vi "MeanderCtrl_3d_StageRefs.vi"(0 "QueuesRef":T1, 1 "MotionStageRefs":refnum<queue>, 2 "AppsRef":refnum<queue>, 3 "SecondaryVI_Ref":refnum<vi>, 4 "SecondaryParams":variant[](array[variant]), 5 "start/end points":cluster{dbl, dbl, dbl}[][](array[cluster]), 9 "Laser_Ctrl":bool, 11 "error in":errorcluster, 12 "HighSpeed":dbl=5.0, 13 "ScanSpeed":dbl=0.1, 14 "KeepStill":u32) -> (6 "Interupted":bool, 8 "Actual_Line#":i32, 15 "error out":errorcluster)   [LabVIEW 2013]
uses:
  ControlDef/QueueRefs.ctl
  ControlDef/LaserCtrl_Method.ctl
  ControlDef/States-AToF.ctl
  <instrlib>/AnalogDiscSDKLv/VIs/DWF_CtrlQueue.ctl
  <instrlib>/AnalogDiscSDKLv/VIs/DWF_State.ctl
  <instrlib>/ESP300/Public/Data/ESP300_State.ctl
  <instrlib>/DG535/Command/DG535_States.ctl
  Hardware/BNC(QuantumComposers)/BNC_States.ctl
  Hardware/FemtoLaser(Legacy)/Laser_Status.ctl
  Hardware/DAQmx(Legacy)/DAQmx_Status.ctl
  ControlDef/Signal.ctl
  ProcessMethods/SignalAverager/ProcessStates.ctl
  Files/WriterState.ctl
  Files/Signal_Segment.ctl
  ControlDef/ProcessingMode.ctl
  Hardware/EPM2000(Legacy)/EPM2K_Status.ctl
  <instrlib>/AnalogDiscSDKLv/VIs/DWF_Signal.ctl
  MeanderLoopState.ctl
  <instrlib>/ESP300/Public/Data/ESP30x_Data.ctl
  <instrlib>/Micos_uic/Public/Data/Micos_Data.ctl
  ControlDef/PauseMeander.vi
  <instrlib>/ESP300/ESP300.lvlib
  <instrlib>/Micos_uic/Micos_uic.lvlib
  <instrlib>/DG535/SRS_DG535_Lib.lvlib
  <userlib>/Utility/ErrorLog_lib.lvlib
  <instrlib>/AnalogDiscSDKLv/AnalogDiscSDKLv.lvlib
panel:
  out "InnerIter.":i32
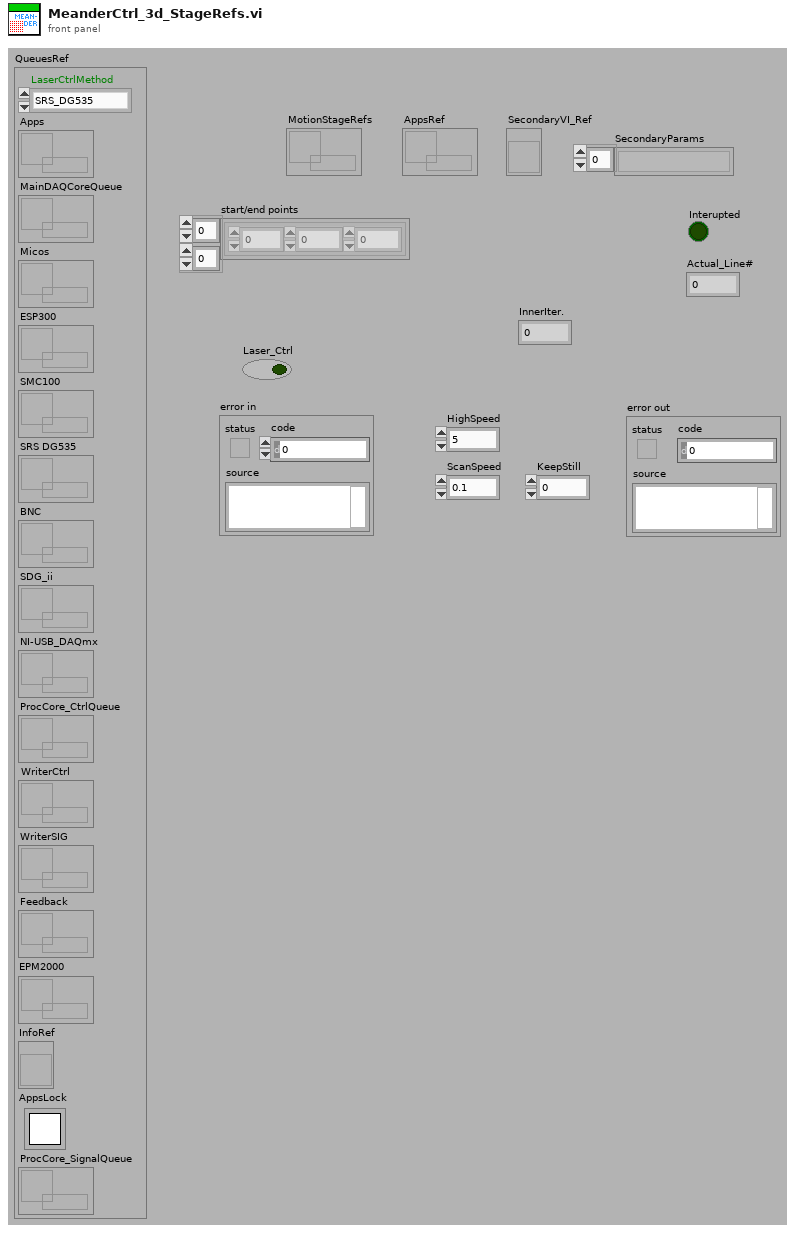
[diagram p1: front panel]
types:
  T1 = typedef "QueueRefs.ctl" = cluster{"LaserCtrlMethod":T2, "Apps":refnum<queue>, "MainDAQCoreQueue":refnum<queue>, "Micos":refnum<queue>, "ESP300":refnum<queue>, "SMC100":refnum<queue>, "SRS DG535":refnum<queue>, "BNC":refnum<queue>, "SDG_ii":refnum<queue>, "NI-USB_DAQmx":refnum<queue>, "ProcCore_CtrlQueue":refnum<queue>, "WriterCtrl":refnum<queue>, "WriterSIG":refnum<queue>, "Feedback":refnum<queue>, "EPM2000":refnum<queue>, "InfoRef":refnum<vi>, "AppsLock":T3, "ProcCore_SignalQueue":refnum<queue>}
  T2 = typedef "LaserCtrl_Method.ctl" = enum16{"SRS_DG535", "BNC", "SDG_II"}
  T3 = typedef "Semaphore RefNum" = refnum<k1>
  T4 = typedef "States-AToF.ctl" = enum16{"Initialize", "Idle", "CalcMzArray", "Meander_SGL_MCS", "Meander_MCS", "CleanSurface", "Meander_Npt", "Meander_SGL_Npt", "KnifeEdgeExpt", "KnifeEdgeExpt_Npt", "Imaging_Micos", "Imaging_ESP", "DepthProfiling", "Set_2PulseDelay", "DelayScan", "PeakSearch", "ExportOrigin", "Save Settings", "Load Settings", "Save as Default", "Load Default", "EnergyCalibration", "Quit", "Interrupted_Stop", "Quit_SubProgram", "StepMove_Joystick", "ContMove_Joystick", "Stop_Joystick", "Check_AppsLock", "Return_Status", "DepthProfile_RT", "UpdateInstruStates", "InstruOptimizer_static", "instruOptimizer_dynamic"}
  T5 = typedef "MeanderLoopState.ctl" = enum16{"Pre-Start", "Send-loginfo", "SetHighVelocity", "MoveToLineStart", "SetSecondaryParams", "WaitStartReady", "UpdateStartPosition", "StartOfLine", "SetLowVelocity", "MoveToLineEnd", "StartLaser_move", "WaitScanFinish", "StartLaser_still", "KeepStill", "StopLaser", "EndOfLine", "CheckPause", "Exit", "RestoreVelocity", "Pause", "Quit"}
  T6 = typedef "ESP300.lvlib/ESP300_State.ctl" = cluster{"State":enum16{"Initialize", "SetDefaultConfig", "Close", "Quit", "Identify", "MoveAbs", "MoveAbs_all", "MoveRel", "MoveRel_all", "STOP", "Origin/Home", "WaitStop", "QueryStatus", "UpdateXPos", "UpdateAll", "SetVelocity", "SetAcceleration", "ClearErr", "LogMessage", "MotorEnable(1)", "EnableAxis", "JoyStick", "GetVelocity", "GetAcceleration", "SendCmd", "SetSoftLimits", "Beep", "_SettingReturn", "SoftReset"}, "Params.":variant}
  T7 = typedef "ESP300.lvlib/ESP30x_Data.ctl" = cluster{"Position":dbl[], "Velocity":dbl[], "Acceleration":dbl[], "Moving":bool, "Simulation":bool, "tickcount_mov":u32, "tickcount_pos":u32, "NumOfAxis":i32, "Initialized":bool, "CommPort":refnum<visa-resource-name>, "Range":dbl[][], "Serial Configuration":cluster{"Baud Rate":u32, "Parity":u16, "Data Bits":u16, "Stop Bits":u16, "Flow Control":u16}, "MotorDisabled":refnum<vi>}
  T8 = typedef "Signal.ctl" = cluster{"Command":T9, "Params":variant}
  T9 = typedef "ProcessStates.ctl" = enum16{"Initialize", "Normal", "Display", "Write2Buffer", "CalcMzArray", "StartSave", "StopSave", "ConfigChanged", "EndOfLine", "SetFilterParams", "SetGraphsEnable", "SetAcquisitionParams", "ChangeDisplayIncrement", "ChangeRepRate", "SetWriterRef", "Quit", "StartOfLine"}
  T10 = typedef "Laser_Status.ctl" = cluster{"State":enum16{"Initialize", "Idle/Update", "Configure", "Turn On", "Tun OFF", "Continuous", "Single Shot", "ManualTrigger", "Close", "Quit"}, "Parameter":dbl}
  T11 = typedef "BNC_States.ctl" = cluster{"State":enum16{"Initialize", "Set System", "Set C-Input", "Set C-Mode", "Set C-Output", "Set C-Enable", "Manl_Trig", "Run", "Stop", "Query C Number", "Close", "Quit"}, "Para.":variant}
  T12 = typedef "SRS_DG535_Lib.lvlib/DG535_States.ctl" = cluster{"State":enum16{"Initialize", "Set Trigger", "Set Output", "Set Delay", "Manl_Trig", "Run", "Stop", "Close", "Quit"}, "Para.":variant}
  T13 = typedef "Micos_uic.lvlib/Micos_Data.ctl" = cluster{"Position":dbl[], "Velocity":dbl[], "Acceleration":dbl[], "Moving":bool, "Simulation":bool, "tickcount_mov":u32, "tickcount_pos":u32, "NumOfAxis":i32, "Initialized":bool, "CommPort":refnum<visa-resource-name>, "Range":dbl[][], "Serial Configuration":cluster{"Baud Rate":u32, "Parity":u16, "Data Bits":u16, "Stop Bits":u16, "Flow Control":u16}, "MotorDisabled":refnum<vi>}
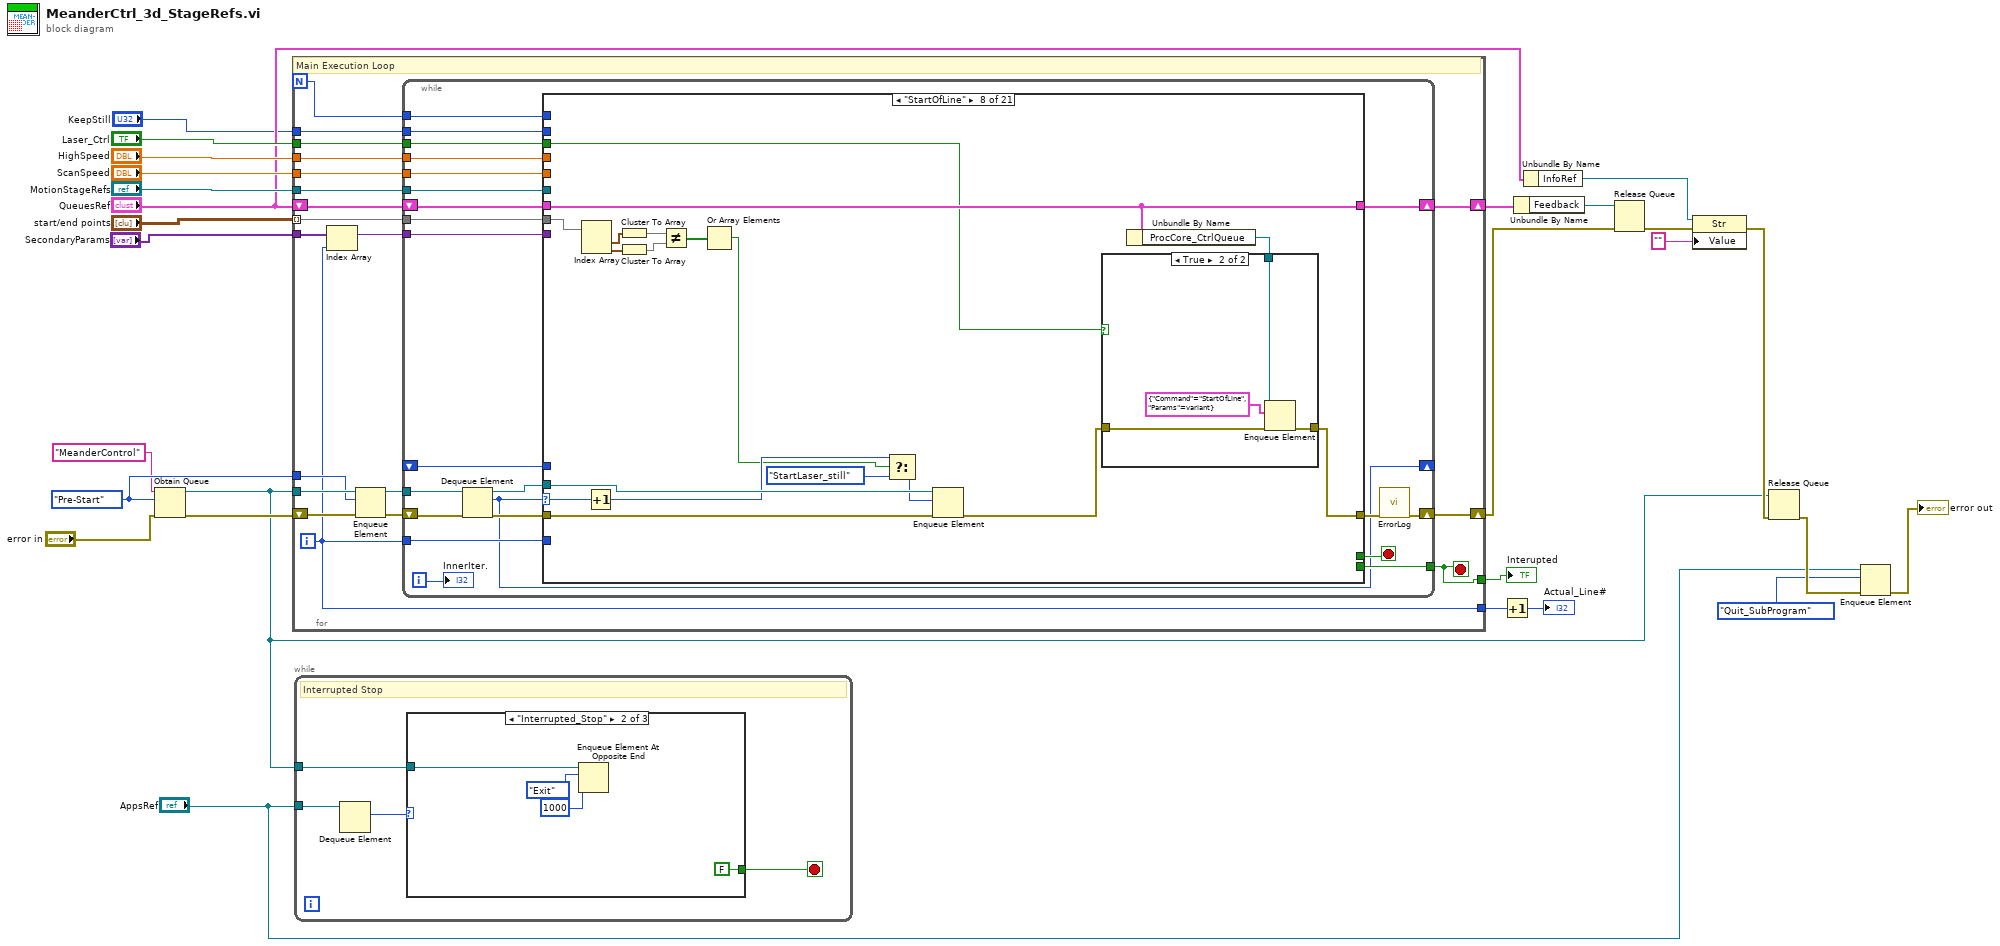
[diagram p0: block diagram]
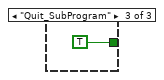
[diagram p3: hidden frame]
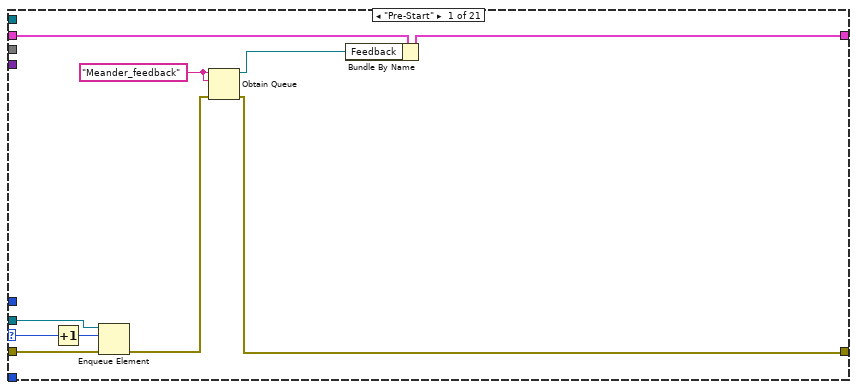
[diagram p4: hidden frame]
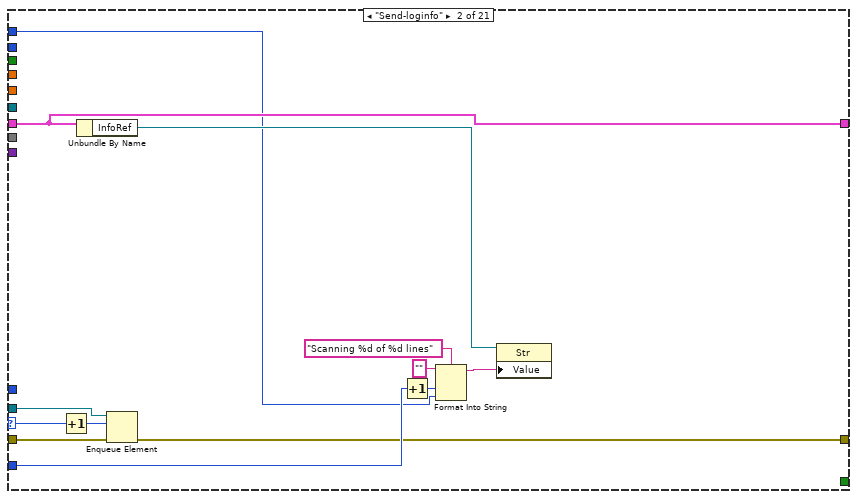
[diagram p5: hidden frame]
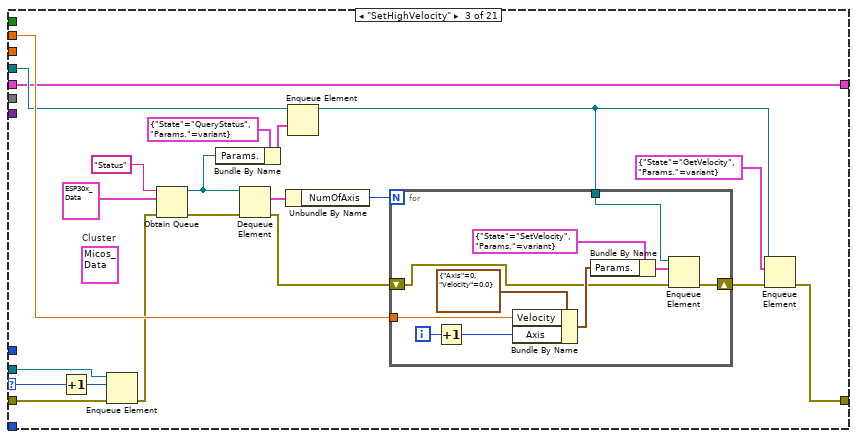
[diagram p6: hidden frame]
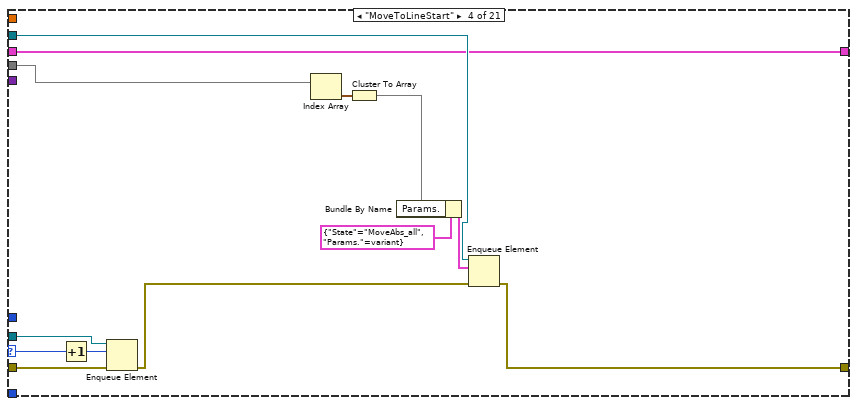
[diagram p7: hidden frame]
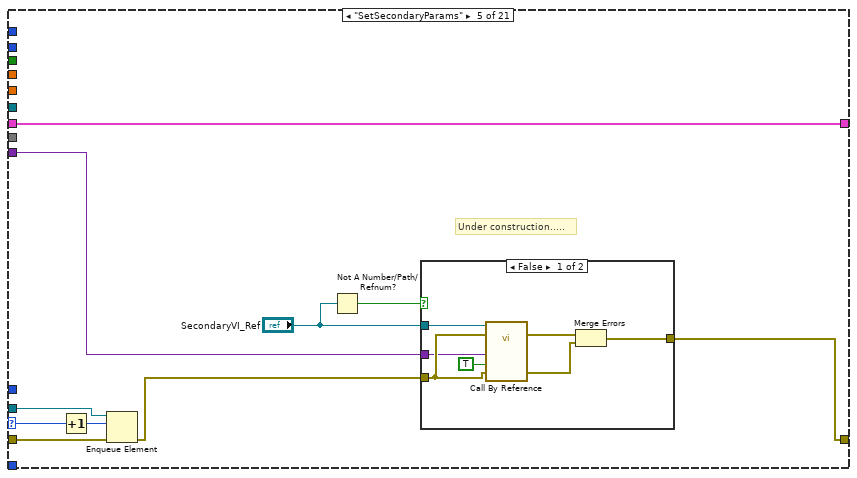
[diagram p8: hidden frame]
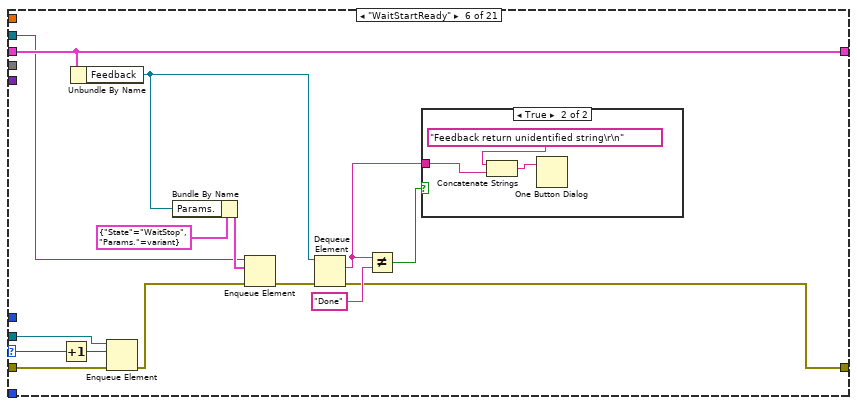
[diagram p10: hidden frame]
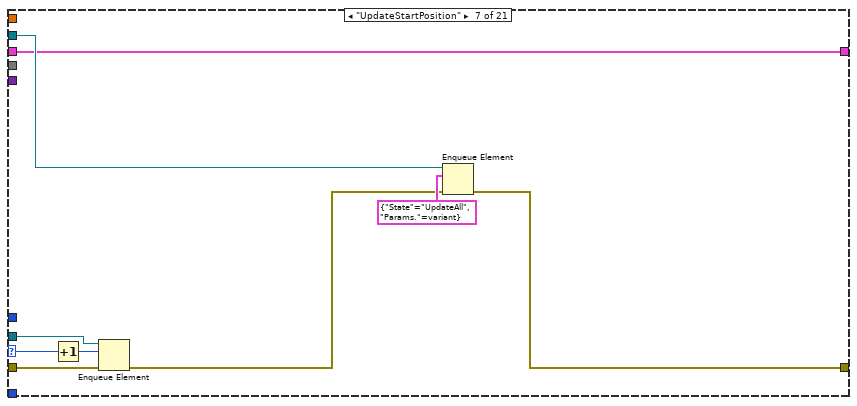
[diagram p12: hidden frame]
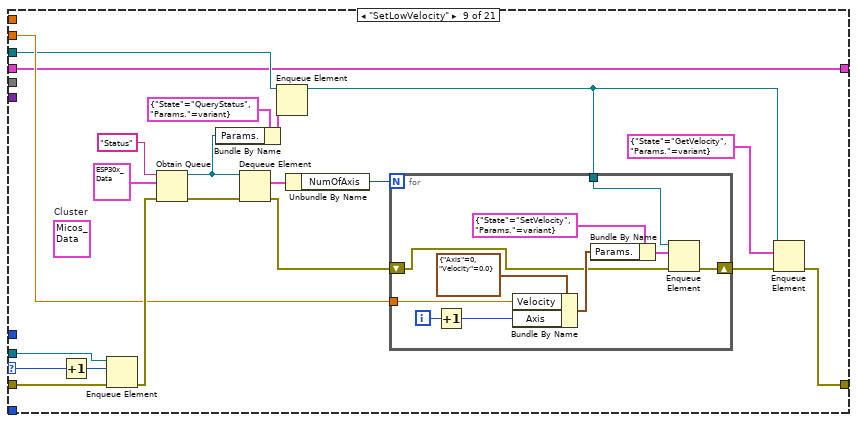
[diagram p14: hidden frame]
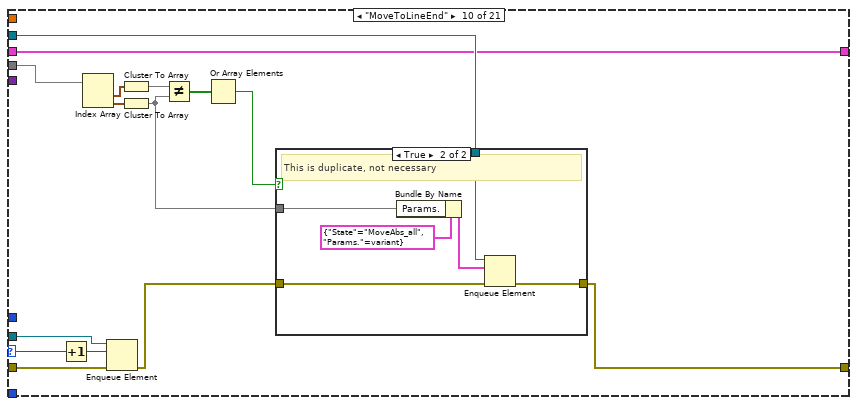
[diagram p15: hidden frame]
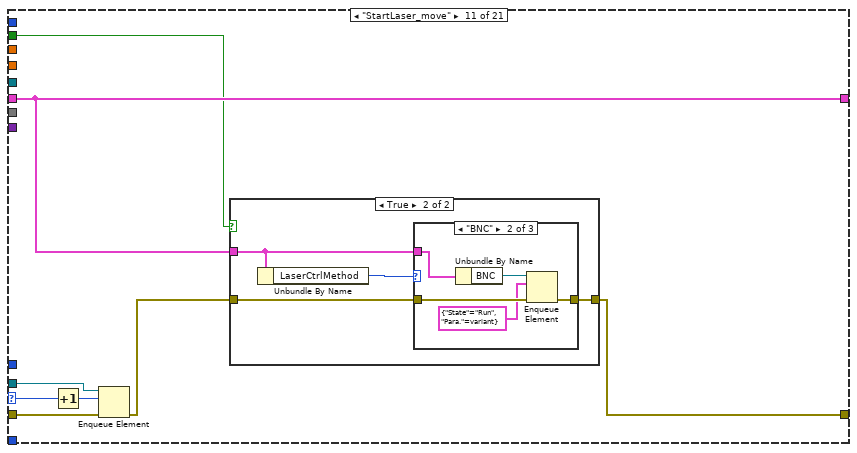
[diagram p17: hidden frame]
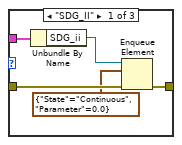
[diagram p19: hidden frame]
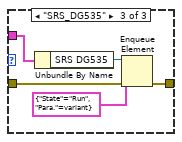
[diagram p20: hidden frame]
diagram:
  w15 = MeanderLoopState."Pre-Start"
  n1 = Obtain Queue(name (unnamed)="MeanderControl", element data type=w15, error in (no error)="error in") -> (queue out=w12:refnum<queue>, error out=w18:errorcluster)  [unwired: 2 in, 1 out]
  n2 = for {
    N -> [w35]
    tunnel: "MotionStageRefs" -> [w45]
    tunnel: "ScanSpeed" -> [w43]
    tunnel: "HighSpeed" -> [w42]
    tunnel: w12 -> [w41]
    tunnel: "start/end points" -> [w40] mode=indexing
    tunnel: "Laser_Ctrl" -> [w39]
    tunnel: [w28] -> w22
    shift-right: [w38] -> w1
    shift-left: w18 -> [w37]
    tunnel: [w36] -> w16
    tunnel: w15 -> [w33]
    shift-right: [w32] -> w3
    shift-left: "QueuesRef" -> [w44]
    tunnel: "KeepStill" -> [w31]
    tunnel: "SecondaryParams" -> [w30]
    i -> [w28]
    stop <- w36 stop-if-true
    # "Main Execution Loop"
    n3 = Index Array(array=w30, index=w28) -> (element=w29:variant)
    n4 = Enqueue Element(queue=w41, element=w33) -> (queue out=w34:refnum<queue>)  [unwired: 2 in, 2 out]
    n5 = while {
      tunnel: w45 -> [w67]
      tunnel: w43 -> [w65]
      tunnel: w42 -> [w64]
      tunnel: w34 -> [w63]
      tunnel: w28 -> [w61]
      shift-right: [w47] -> w38
      shift-left: w37 -> [w58]
      tunnel: w40 -> [w56]
      tunnel: w39 -> [w55]
      shift-right: [w46] -> _
      shift-left: _ -> [w54]
      tunnel: [w53] -> w36
      tunnel: w35 -> [w52]
      shift-right: [w51] -> w32
      shift-left: w44 -> [w66]
      tunnel: w31 -> [w50]
      tunnel: w29 -> [w48]
      i -> [w49]
      stop <- w62 stop-if-true
      n6 = Dequeue Element(queue=w63, error in (no error)=w58) -> (queue out=w60:refnum<queue>, element=w46:T5, error out=w59:errorcluster)  [unwired: 1 in, 1 out]
      n7 = case shown="\"StartOfLine\"" w46 {
        selector: w46 -> [w77 w90 w111 w134 w144 w167 w179 w197 w223 w248 w263 w298 w312 w340 w365 _ _ _ _ _ _]
        tunnel: w67 -> [_ _ w97 w123 _ w153 w174 _ w210 w240 _ w284 _ _ _ _ w410 _ w468 _ _]
        tunnel: w66 -> [w71 w85 w96 w122 w140 w165 w171 w194 w209 w239 w259 w296 w304 w336 w360 w392 w409 w440 w461 w470 w500]
        tunnel: w65 -> [_ _ _ _ _ _ _ _ w211 _ _ _ _ _ _ _ _ _ _ _ _]
        tunnel: w64 -> [_ _ w107 _ _ _ _ _ _ _ _ _ _ _ _ _ w421 _ _ _ _]
        tunnel: [_ _ _ _ _ _ _ _ _ _ _ _ _ _ _ _ w400 TRUE _ _ w499] -> w62
        tunnel: w61 -> [_ w83 _ _ _ _ _ _ _ _ _ _ _ _ _ _ _ _ _ _ _]
        tunnel: w60 -> [w72 w82 w109 w132 w142 w164 w177 w196 w221 w246 w261 w295 w310 w333 w363 w394 w407 w439 w458 w474 _]
        tunnel: w59 -> [w75 w81 w108 w131 w141 w163 w176 w195 w220 w245 w260 w294 w309 w338 w362 w393 w406 w442 w469 w477 w498]
        tunnel: [w73 w80 w91 w124 w138 w154 w172 w191 w204 w242 w256 w285 w302 w337 w358 w389 w412 w438 _ w476 w498] -> w57
        tunnel: w56 -> [_ _ _ w128 _ _ _ w183 _ w244 _ _ _ _ _ _ _ _ _ _ _]
        tunnel: w55 -> [_ _ _ _ _ _ _ w190 _ _ w258 _ w308 _ w361 w388 _ _ _ _ _]
        tunnel: w54 -> [_ _ _ _ _ _ _ _ _ _ _ _ _ _ _ _ w404 _ _ _ _]
        tunnel: [_ _ _ _ _ _ _ _ _ _ _ _ _ _ _ _ w401 w441 _ _ w499] -> w53
        tunnel: w52 -> [_ w78 _ _ _ _ _ _ _ _ _ _ _ _ _ _ _ _ _ _ _]
        tunnel: [w70 w85 w96 w122 w140 w165 w171 w194 w209 w239 w259 w296 w304 w336 w360 w392 w409 w440 w461 w470 w500] -> w51
        tunnel: w50 -> [_ _ _ _ _ _ _ _ _ _ _ _ w307 w335 _ _ _ _ _ _ _]
        tunnel: w48 -> [_ _ _ _ w135 _ _ _ _ _ _ _ _ _ _ _ _ _ _ _ _]
        frame "Pre-Start" {
          w68 = "Meander_feedback" ("name (unnamed)")
          n8 = Increment(x=w77) -> (x+1=w76:T5)
          n9 = Enqueue Element(queue=w72, element=w76, error in (no error)=w75) -> (error out=w74:errorcluster)  [unwired: 1 in, 2 out]
          n10 = Obtain Queue(name (unnamed)=w68, element data type=w68, error in (no error)=w74) -> (queue out=w69:refnum<queue>, error out=w73:errorcluster)  [unwired: 2 in, 1 out]
          n11 = Bundle By Name(cluster=w71, "Feedback"=w69) -> (w70:T1)
        }
        frame "Send-loginfo" {
          n12 = Increment(x=w90) -> (x+1=w89:T5)
          n13 = Unbundle By Name(w85) -> ("InfoRef"=w84:refnum<vi>)
          n14 = Enqueue Element(queue=w82, element=w89, error in (no error)=w81) -> (error out=w80:errorcluster)  [unwired: 1 in, 2 out]
          n15 = Increment(x=w83) -> (x+1=w87:i32)
          n16 = Format Into String(format string="Scanning %d of %d lines", initial string="", w87, w78) -> (resulting string=w88:string)  [unwired: 1 in, 1 out]
          n17 = property class="Str"(reference=w84, "Value"=w88) -> ()  [unwired: 1 in, 2 out]
        }
        frame "SetHighVelocity" {
          (unwired) T13 {"Position"=[], "Velocity"=[], "Acceleration"=[], "Moving"=FALSE, "Simulation"=FALSE, "tickcount_mov"=0, "tickcount_pos"=0, "NumOfAxis"=0, "Initialized"=FALSE, "CommPort"="", "Range"=[], "Serial Configuration"={"Baud Rate"=19200, "Parity"=0, "Data Bits"=8, "Stop Bits"=10, "Flow Control"=0}, "MotorDisabled"=refnum}  # Cluster
          n18 = Increment(x=w111) -> (x+1=w110:T5)
          n19 = Enqueue Element(queue=w109, element=w110, error in (no error)=w108) -> (error out=w99:errorcluster)  [unwired: 1 in, 2 out]
          n20 = Obtain Queue(name (unnamed)="Status", element data type=T7 {"Position"=[], "Velocity"=[], "Acceleration"=[], "Moving"=FALSE, "Simulation"=FALSE, "tickcount_mov"=0, "tickcount_pos"=0, "NumOfAxis"=0, "Initialized"=FALSE, "CommPort"="", "Range"=[], "Serial Configuration"={"Baud Rate"=0, "Parity"=0, "Data Bits"=0, "Stop Bits"=0, "Flow Control"=0}, "MotorDisabled"=refnum}, error in (no error)=w99) -> (queue out=w104:refnum<queue>, error out=w103:errorcluster)  [unwired: 2 in, 1 out]
          n21 = Bundle By Name(cluster=T6 {"State"=enum."QueryStatus", "Params."=variant} ("element"), "Params."=w104) -> (w105:T6)
          n22 = Dequeue Element(queue=w104, error in (no error)=w103) -> (element=w102:T7, error out=w100:errorcluster)  [unwired: 1 in, 2 out]
          n23 = Unbundle By Name(w102) -> ("NumOfAxis"=w101:i32)
          n24 = Enqueue Element(queue=w97, element=w105) -> (queue out=w93:refnum<queue>)  [unwired: 2 in, 2 out]
          n25 = for {
            N: w101 -> [_]
            tunnel: w93 -> [w115]
            tunnel: w107 -> [w114]
            shift-right: [w112] -> w94
            shift-left: w100 -> [w113]
            i -> [w121]
            n26 = Increment(x=w121) -> (x+1=w119:i32)
            n27 = Bundle By Name(cluster=cluster{"Axis":i32, "Velocity":dbl} {"Axis"=0, "Velocity"=0.0}, "Velocity"=w114, "Axis"=w119) -> (w116:cluster{"Axis":i32, "Velocity":dbl})
            n28 = Bundle By Name(cluster=T6 {"State"=enum."SetVelocity", "Params."=variant} ("element"), "Params."=w116) -> (w118:T6)
            n29 = Enqueue Element(queue=w115, element=w118, error in (no error)=w113) -> (error out=w112:errorcluster)  [unwired: 1 in, 2 out]
          }
          n30 = Enqueue Element(queue=w93, element=T6 {"State"=enum."GetVelocity", "Params."=variant}, error in (no error)=w94) -> (error out=w91:errorcluster)  [unwired: 1 in, 2 out]
        }
        frame "MoveToLineStart" {
          n31 = Increment(x=w134) -> (x+1=w133:T5)
          n32 = Enqueue Element(queue=w132, element=w133, error in (no error)=w131) -> (error out=w125:errorcluster)  [unwired: 1 in, 2 out]
          n33 = Index Array(array=w128) -> (element=w127:cluster{dbl, dbl, dbl})  [unwired: 1 in]
          n34 = Cluster To Array(cluster=w127) -> (array=w126:dbl[])
          n35 = Bundle By Name(cluster=T6 {"State"=enum."MoveAbs_all", "Params."=variant} ("element"), "Params."=w126) -> (w129:T6)
          n36 = Enqueue Element(queue=w123, element=w129, error in (no error)=w125) -> (error out=w124:errorcluster)  [unwired: 1 in, 2 out]
        }
        frame "SetSecondaryParams" {
          # "Under construction....."
          n37 = Increment(x=w144) -> (x+1=w143:T5)
          n38 = Enqueue Element(queue=w142, element=w143, error in (no error)=w141) -> (error out=w139:errorcluster)  [unwired: 1 in, 2 out]
          n39 = Not A Number/Path/Refnum?(number/path/refnum="SecondaryVI_Ref") -> (NaN/Path/Refnum?=w137:bool)
          n40 = case shown="False" w137 {
            tunnel: w139 -> [w151 w152]
            tunnel: [w150 w152] -> w138
            tunnel: "SecondaryVI_Ref" -> [w149 _]
            tunnel: w135 -> [w145 _]
            frame False {
              n41 = call-by-ref "?"(reference=w149, error in=w151, "error in"=w151, "WaitForReady"=TRUE, "InputParams."=w145) -> (error out=w148:errorcluster, 0:"error out"=w147:errorcluster)  [unwired: 7 in, 2 out]
              n42 = Merge Errors(w148, w147) -> (w150:errorcluster)
            }
            frame True {
            }
          }
        }
        frame "WaitStartReady" {
          n43 = Increment(x=w167) -> (x+1=w166:T5)
          n44 = Unbundle By Name(w165) -> ("Feedback"=w158:refnum<queue>)
          n45 = Enqueue Element(queue=w164, element=w166, error in (no error)=w163) -> (error out=w160:errorcluster)  [unwired: 1 in, 2 out]
          n46 = Bundle By Name(cluster=T6 {"State"=enum."WaitStop", "Params."=variant} ("element"), "Params."=w158) -> (w161:T6)
          n47 = Enqueue Element(queue=w153, element=w161, error in (no error)=w160) -> (error out=w159:errorcluster)  [unwired: 1 in, 2 out]
          n48 = Dequeue Element(queue=w158, error in (no error)=w159) -> (element=w155:string, error out=w154:errorcluster)  [unwired: 1 in, 2 out]
          n49 = Not Equal?(x=w155, y="Done" ("element")) -> (x != y?=w156:bool)
          n50 = case shown="True" w156 {
            tunnel: w155 -> [_ w168]
            frame False {
            }
            frame True {
              n51 = Concatenate Strings("Feedback return unidentified string\r\n" ("message"), w168) -> (w169:string)
              n52 = One Button Dialog(message=w169) -> ()  [unwired: 1 in, 1 out]
            }
          }
        }
        frame "UpdateStartPosition" {
          n53 = Increment(x=w179) -> (x+1=w178:T5)
          n54 = Enqueue Element(queue=w177, element=w178, error in (no error)=w176) -> (error out=w173:errorcluster)  [unwired: 1 in, 2 out]
          n55 = Enqueue Element(queue=w174, element=T6 {"State"=enum."UpdateAll", "Params."=variant}, error in (no error)=w173) -> (error out=w172:errorcluster)  [unwired: 1 in, 2 out]
        }
        frame "StartOfLine" {
          n56 = Index Array(array=w183) -> (element #1=w187:cluster{dbl, dbl, dbl}, element #2=w188:cluster{dbl, dbl, dbl})  [unwired: 2 in]
          n57 = Increment(x=w197) -> (x+1=w182:T5)
          n58 = Cluster To Array(cluster=w187) -> (array=w186:dbl[])
          n59 = Cluster To Array(cluster=w188) -> (array=w185:dbl[])
          n60 = Not Equal?(x=w186, y=w185) -> (x != y?=w184:bool[])
          n61 = Or Array Elements(Boolean array=w184) -> (logical OR=w180:bool)
          n62 = Select(t=w182, s=w180, f=MeanderLoopState."StartLaser_still") -> (s? t:f=w189:T5)
          n63 = Enqueue Element(queue=w196, element=w189, error in (no error)=w195) -> (error out=w192:errorcluster)  [unwired: 1 in, 2 out]
          n64 = Unbundle By Name(w194) -> ("ProcCore_CtrlQueue"=w193:refnum<queue>)
          n65 = case shown="True" w190 {
            tunnel: w192 -> [w198 w202]
            tunnel: [w198 w201] -> w191
            tunnel: w193 -> [_ w200]
            frame False {
            }
            frame True {
              n66 = Enqueue Element(queue=w200, element=T8 {"Command"=enum."StartOfLine", "Params"=variant}, error in (no error)=w202) -> (error out=w201:errorcluster)  [unwired: 1 in, 2 out]
            }
          }
        }
        frame "SetLowVelocity" {
          (unwired) T13 {"Position"=[], "Velocity"=[], "Acceleration"=[], "Moving"=FALSE, "Simulation"=FALSE, "tickcount_mov"=0, "tickcount_pos"=0, "NumOfAxis"=0, "Initialized"=FALSE, "CommPort"="", "Range"=[], "Serial Configuration"={"Baud Rate"=19200, "Parity"=0, "Data Bits"=8, "Stop Bits"=10, "Flow Control"=0}, "MotorDisabled"=refnum}  # Cluster
          n67 = Increment(x=w223) -> (x+1=w222:T5)
          n68 = Enqueue Element(queue=w221, element=w222, error in (no error)=w220) -> (error out=w212:errorcluster)  [unwired: 1 in, 2 out]
          n69 = Obtain Queue(name (unnamed)="Status", element data type=T7 {"Position"=[], "Velocity"=[], "Acceleration"=[], "Moving"=FALSE, "Simulation"=FALSE, "tickcount_mov"=0, "tickcount_pos"=0, "NumOfAxis"=0, "Initialized"=FALSE, "CommPort"="", "Range"=[], "Serial Configuration"={"Baud Rate"=0, "Parity"=0, "Data Bits"=0, "Stop Bits"=0, "Flow Control"=0}, "MotorDisabled"=refnum}, error in (no error)=w212) -> (queue out=w217:refnum<queue>, error out=w216:errorcluster)  [unwired: 2 in, 1 out]
          n70 = Bundle By Name(cluster=T6 {"State"=enum."QueryStatus", "Params."=variant} ("element"), "Params."=w217) -> (w218:T6)
          n71 = Dequeue Element(queue=w217, error in (no error)=w216) -> (element=w215:T7, error out=w213:errorcluster)  [unwired: 1 in, 2 out]
          n72 = Enqueue Element(queue=w210, element=w218) -> (queue out=w206:refnum<queue>)  [unwired: 2 in, 2 out]
          n73 = Unbundle By Name(w215) -> ("NumOfAxis"=w214:i32)
          n74 = for {
            N: w214 -> [_]
            tunnel: w206 -> [w227]
            tunnel: w211 -> [w226]
            shift-right: [w224] -> w205
            shift-left: w213 -> [w225]
            i -> [w233]
            n75 = Increment(x=w233) -> (x+1=w231:i32)
            n76 = Bundle By Name(cluster=cluster{"Axis":i32, "Velocity":dbl} {"Axis"=0, "Velocity"=0.0}, "Velocity"=w226, "Axis"=w231) -> (w228:cluster{"Axis":i32, "Velocity":dbl})
            n77 = Bundle By Name(cluster=T6 {"State"=enum."SetVelocity", "Params."=variant} ("element"), "Params."=w228) -> (w230:T6)
            n78 = Enqueue Element(queue=w227, element=w230, error in (no error)=w225) -> (error out=w224:errorcluster)  [unwired: 1 in, 2 out]
          }
          n79 = Enqueue Element(queue=w206, element=T6 {"State"=enum."GetVelocity", "Params."=variant}, error in (no error)=w205) -> (error out=w204:errorcluster)  [unwired: 1 in, 2 out]
        }
        frame "MoveToLineEnd" {
          n80 = Increment(x=w248) -> (x+1=w247:T5)
          n81 = Index Array(array=w244) -> (element #1=w238:cluster{dbl, dbl, dbl}, element #2=w241:cluster{dbl, dbl, dbl})  [unwired: 2 in]
          n82 = Enqueue Element(queue=w246, element=w247, error in (no error)=w245) -> (error out=w243:errorcluster)  [unwired: 1 in, 2 out]
          n83 = Cluster To Array(cluster=w238) -> (array=w237:dbl[])
          n84 = Cluster To Array(cluster=w241) -> (array=w236:dbl[])
          n85 = Not Equal?(x=w237, y=w236) -> (x != y?=w235:bool[])
          n86 = Or Array Elements(Boolean array=w235) -> (logical OR=w234:bool)
          n87 = case shown="True" w234 {
            tunnel: w243 -> [w249 w253]
            tunnel: [w249 w252] -> w242
            tunnel: w240 -> [_ w251]
            tunnel: w236 -> [_ w250]
            frame False {
            }
            frame True {
              # "This is duplicate, not necessary"
              n88 = Bundle By Name(cluster=T6 {"State"=enum."MoveAbs_all", "Params."=variant} ("element"), "Params."=w250) -> (w254:T6)
              n89 = Enqueue Element(queue=w251, element=w254, error in (no error)=w253) -> (error out=w252:errorcluster)  [unwired: 1 in, 2 out]
            }
          }
        }
        frame "StartLaser_move" {
          n90 = Increment(x=w263) -> (x+1=w262:T5)
          n91 = Enqueue Element(queue=w261, element=w262, error in (no error)=w260) -> (error out=w257:errorcluster)  [unwired: 1 in, 2 out]
          n92 = case shown="True" w258 {
            tunnel: [w264 w268] -> w256
            tunnel: w257 -> [w264 w267]
            tunnel: w259 -> [_ w266]
            frame False {
            }
            frame True {
              n93 = Unbundle By Name(w266) -> ("LaserCtrlMethod"=w265:T2)
              n94 = case shown="\"BNC\"" w265 {
                tunnel: [w273 w278 w283] -> w268
                tunnel: w267 -> [w272 w277 w282]
                tunnel: w266 -> [w270 w276 w281]
                frame "SDG_II" {
                  n95 = Unbundle By Name(w270) -> ("SDG_ii"=w269:refnum<queue>)
                  n96 = Enqueue Element(queue=w269, element=T10 {"State"=enum."Continuous", "Parameter"=0.0}, error in (no error)=w272) -> (error out=w273:errorcluster)  [unwired: 1 in, 2 out]
                }
                frame "BNC" {
                  n97 = Unbundle By Name(w276) -> ("BNC"=w275:refnum<queue>)
                  n98 = Enqueue Element(queue=w275, element=T11 {"State"=enum."Run", "Para."=variant}, error in (no error)=w277) -> (error out=w278:errorcluster)  [unwired: 1 in, 2 out]
                }
                frame "SRS_DG535" {
                  n99 = Unbundle By Name(w281) -> ("SRS DG535"=w280:refnum<queue>)
                  n100 = Enqueue Element(queue=w280, element=T12 {"State"=enum."Run", "Para."=variant}, error in (no error)=w282) -> (error out=w283:errorcluster)  [unwired: 1 in, 2 out]
                }
              }
            }
          }
        }
        frame "WaitScanFinish" {
          n101 = Increment(x=w298) -> (x+1=w297:T5)
          n102 = Unbundle By Name(w296) -> ("Feedback"=w289:refnum<queue>)
          n103 = Enqueue Element(queue=w295, element=w297, error in (no error)=w294) -> (error out=w291:errorcluster)  [unwired: 1 in, 2 out]
          n104 = Bundle By Name(cluster=T6 {"State"=enum."WaitStop", "Params."=variant} ("element"), "Params."=w289) -> (w292:T6)
          n105 = Enqueue Element(queue=w284, element=w292, error in (no error)=w291) -> (error out=w290:errorcluster)  [unwired: 1 in, 2 out]
          n106 = Dequeue Element(queue=w289, error in (no error)=w290) -> (element=w286:string, error out=w285:errorcluster)  [unwired: 1 in, 2 out]
          n107 = Not Equal?(x=w286, y="Done" ("element")) -> (x != y?=w287:bool)
          n108 = case shown="True" w287 {
            tunnel: w286 -> [_ w299]
            frame False {
            }
            frame True {
              n109 = Concatenate Strings("WaitStop Feedback return unidentified string\r\n" ("message"), w299) -> (w300:string)
              n110 = One Button Dialog(message=w300) -> ()  [unwired: 1 in, 1 out]
            }
          }
        }
        frame "StartLaser_still" {
          n111 = Increment(x=w312) -> (x+1=w311:T5)
          n112 = Enqueue Element(queue=w310, element=w311, error in (no error)=w309) -> (error out=w303:errorcluster)  [unwired: 1 in, 2 out]
          n113 = Not Equal To 0?(x=w307) -> (x != 0?=w306:bool)
          n114 = And(x=w306, y=w308) -> (x .and. y?=w305:bool)
          n115 = case shown="True" w305 {
            tunnel: [w313 w317] -> w302
            tunnel: w303 -> [w313 w316]
            tunnel: w304 -> [_ w315]
            frame False {
            }
            frame True {
              n116 = Unbundle By Name(w315) -> ("LaserCtrlMethod"=w314:T2)
              n117 = case shown="\"BNC\"" w314 {
                tunnel: [w322 w327 w332] -> w317
                tunnel: w316 -> [w321 w326 w331]
                tunnel: w315 -> [w319 w325 w330]
                frame "SDG_II" {
                  n118 = Unbundle By Name(w319) -> ("SDG_ii"=w318:refnum<queue>)
                  n119 = Enqueue Element(queue=w318, element=T10 {"State"=enum."Continuous", "Parameter"=0.0}, error in (no error)=w321) -> (error out=w322:errorcluster)  [unwired: 1 in, 2 out]
                }
                frame "BNC" {
                  n120 = Unbundle By Name(w325) -> ("BNC"=w324:refnum<queue>)
                  n121 = Enqueue Element(queue=w324, element=T11 {"State"=enum."Run", "Para."=variant}, error in (no error)=w326) -> (error out=w327:errorcluster)  [unwired: 1 in, 2 out]
                }
                frame "SRS_DG535" {
                  n122 = Unbundle By Name(w330) -> ("SRS DG535"=w329:refnum<queue>)
                  n123 = Enqueue Element(queue=w329, element=T12 {"State"=enum."Run", "Para."=variant}, error in (no error)=w331) -> (error out=w332:errorcluster)  [unwired: 1 in, 2 out]
                }
              }
            }
          }
        }
        frame "KeepStill" {
          n124 = case shown="Default" w335 {
            selector: w335 -> [_ w343]
            tunnel: [w341 w346] -> w334
            tunnel: w333 -> [w341 w345]
            frame 0 {
            }
            frame Default {
              # "Enable emergency interrupt exit"
              n125 = Tick Count (ms)() -> (millisecond timer value=w344:u32)
              n126 = Add(x=w344, y=w343) -> (x+y=w342:u32)
              n127 = while {
                tunnel: [w357] -> w346
                tunnel: w345 -> [w356]
                tunnel: w342 -> [w351]
                stop <- w348 stop-if-true
                n128 = Wait (ms)(milliseconds to wait=u32 1) -> ()  [unwired: 1 out]
                n129 = Tick Count (ms)() -> (millisecond timer value=w350:u32)
                n130 = Preview Queue Element(queue=w356, timeout in ms (-1)=0) -> (queue out=w357:refnum<queue>, element=w353:T5)  [unwired: 1 in, 2 out]
                n131 = Equal?(x=w353, y=MeanderLoopState."Exit" ("element")) -> (x = y?=w352:bool)
                n132 = Greater?(x=w350, y=w351) -> (0:w349:bool)
                n133 = Or(x=w349, y=w352) -> (x .or. y?=w348:bool)
              }
            }
          }
          n134 = Increment(x=w340) -> (x+1=w339:T5)
          n135 = Enqueue Element(queue=w334, element=w339, error in (no error)=w338) -> (error out=w337:errorcluster)  [unwired: 1 in, 2 out]
        }
        frame "StopLaser" {
          n136 = Increment(x=w365) -> (x+1=w364:T5)
          n137 = Enqueue Element(queue=w363, element=w364, error in (no error)=w362) -> (error out=w359:errorcluster)  [unwired: 1 in, 2 out]
          n138 = case shown="True" w361 {
            tunnel: [w366 w371] -> w358
            tunnel: w359 -> [w366 w370]
            tunnel: w360 -> [_ w369]
            frame False {
            }
            frame True {
              n139 = Unbundle By Name(w369) -> ("LaserCtrlMethod"=w368:T2)
              n140 = case shown="\"SRS_DG535\"" w368 {
                tunnel: [w376 w381 w386] -> w371
                tunnel: w370 -> [w375 w380 w385]
                tunnel: w369 -> [w373 w379 w384]
                frame "SDG_II" {
                  n141 = Unbundle By Name(w373) -> ("SDG_ii"=w372:refnum<queue>)
                  n142 = Enqueue Element(queue=w372, element=T10 {"State"=enum."Single Shot", "Parameter"=0.0}, error in (no error)=w375) -> (error out=w376:errorcluster)  [unwired: 1 in, 2 out]
                }
                frame "BNC" {
                  n143 = Unbundle By Name(w379) -> ("BNC"=w378:refnum<queue>)
                  n144 = Enqueue Element(queue=w378, element=T11 {"State"=enum."Stop", "Para."=variant}, error in (no error)=w380) -> (error out=w381:errorcluster)  [unwired: 1 in, 2 out]
                }
                frame "SRS_DG535" {
                  n145 = Unbundle By Name(w384) -> ("SRS DG535"=w383:refnum<queue>)
                  n146 = Enqueue Element(queue=w383, element=T12 {"State"=enum."Stop", "Para."=variant}, error in (no error)=w385) -> (error out=w386:errorcluster)  [unwired: 1 in, 2 out]
                }
              }
              n147 = Wait (ms) "Wait for laser actually stop"(milliseconds to wait=u32 50) -> ()  [unwired: 1 out]
            }
          }
        }
        frame "EndOfLine" {
          n148 = Enqueue Element(queue=w394, element=MeanderLoopState."RestoreVelocity", error in (no error)=w393) -> (error out=w390:errorcluster)  [unwired: 1 in, 2 out]
          n149 = Unbundle By Name(w392) -> ("ProcCore_CtrlQueue"=w391:refnum<queue>)
          n150 = case shown="True" w388 {
            tunnel: w390 -> [w395 w399]
            tunnel: [w395 w398] -> w389
            tunnel: w391 -> [_ w397]
            frame False {
            }
            frame True {
              n151 = Enqueue Element(queue=w397, element=T8 {"Command"=enum."EndOfLine", "Params"=variant}, error in (no error)=w399) -> (error out=w398:errorcluster)  [unwired: 1 in, 2 out]
            }
          }
        }
        frame "RestoreVelocity" {
          (unwired) T13 {"Position"=[], "Velocity"=[], "Acceleration"=[], "Moving"=FALSE, "Simulation"=FALSE, "tickcount_mov"=0, "tickcount_pos"=0, "NumOfAxis"=0, "Initialized"=FALSE, "CommPort"="", "Range"=[], "Serial Configuration"={"Baud Rate"=19200, "Parity"=0, "Data Bits"=8, "Stop Bits"=10, "Flow Control"=0}, "MotorDisabled"=refnum}  # Cluster
          n152 = Equal?(x=MeanderLoopState."Quit" ("element"), y=w404) -> (x = y?=w403:bool)
          n153 = case shown="False" w403 {
            tunnel: w407 -> [w425 _]
            tunnel: w406 -> [w424 w427]
            tunnel: [w422 w427] -> w402
            tunnel: [_ w426] -> w401
            tunnel: [_ w426] -> w400
            frame False {
              n154 = Enqueue Element(queue=w425, element=MeanderLoopState."CheckPause", error in (no error)=w424) -> (error out=w422:errorcluster)  [unwired: 1 in, 2 out]
            }
            frame True {
              w426 = TRUE
            }
          }
          n155 = Obtain Queue(name (unnamed)="Status", element data type=T7 {"Position"=[], "Velocity"=[], "Acceleration"=[], "Moving"=FALSE, "Simulation"=FALSE, "tickcount_mov"=0, "tickcount_pos"=0, "NumOfAxis"=0, "Initialized"=FALSE, "CommPort"="", "Range"=[], "Serial Configuration"={"Baud Rate"=0, "Parity"=0, "Data Bits"=0, "Stop Bits"=0, "Flow Control"=0}, "MotorDisabled"=refnum}, error in (no error)=w402) -> (queue out=w417:refnum<queue>, error out=w416:errorcluster)  [unwired: 2 in, 1 out]
          n156 = Bundle By Name(cluster=T6 {"State"=enum."QueryStatus", "Params."=variant} ("element"), "Params."=w417) -> (w418:T6)
          n157 = Dequeue Element(queue=w417, error in (no error)=w416) -> (element=w415:T7, error out=w413:errorcluster)  [unwired: 1 in, 2 out]
          n158 = Enqueue Element(queue=w410, element=w418) -> (queue out=w420:refnum<queue>)  [unwired: 2 in, 2 out]
          n159 = Unbundle By Name(w415) -> ("NumOfAxis"=w414:i32)
          n160 = for {
            N: w414 -> [_]
            tunnel: w420 -> [w431]
            tunnel: w421 -> [w430]
            shift-right: [w428] -> w412
            shift-left: w413 -> [w429]
            i -> [w437]
            n161 = Increment(x=w437) -> (x+1=w435:i32)
            n162 = Bundle By Name(cluster=cluster{"Axis":i32, "Velocity":dbl} {"Axis"=0, "Velocity"=0.0}, "Velocity"=w430, "Axis"=w435) -> (w432:cluster{"Axis":i32, "Velocity":dbl})
            n163 = Bundle By Name(cluster=T6 {"State"=enum."SetVelocity", "Params."=variant} ("element"), "Params."=w432) -> (w434:T6)
            n164 = Enqueue Element(queue=w431, element=w434, error in (no error)=w429) -> (error out=w428:errorcluster)  [unwired: 1 in, 2 out]
          }
        }
        frame "CheckPause" {
          n165 = while {
            shift-right: [w447] -> w438
            shift-left: w442 -> [w454]
            tunnel: w439 -> [w455]
            tunnel: [w445] -> w441
            stop <- w451 continue-if-true
            n166 = Preview Queue Element(queue=w455, timeout in ms (-1)=0, error in (no error)=w454) -> (element=w452:T5, timed out?=w449:bool, error out=w448:errorcluster)  [unwired: 1 out]
            n167 = global read "PauseMeander.vi" "Pause Meaner"() -> (w456:bool)
            n168 = Not Equal?(x=MeanderLoopState."Exit", y=w452) -> (x != y?=w450:bool)
            n169 = Compound Arithmetic op=AND(w450, invert w449) -> (w445:bool)
            n170 = Not(x=w445) -> (.not. x?=w444:bool)
            n171 = Or(x=w456, y=w445) -> (x .or. y?=w451:bool)
            n172 = call <userlib>:"Wait (ms)__ogtk.vi"("error in (no error)"=w448, "Wait on Error (FALSE)"=w444, "milliseconds to wait"=u32 200) -> ("error out"=w447:errorcluster)  [unwired: 7 in, 1 out]
          }
        }
        frame "Exit" {
          # "Next frame: \nrestore high velocity"
          # "Stop stage\nstop laser\nrestore high velocity\nexit"
          n173 = Enqueue Element At Opposite End(queue=w458, element=MeanderLoopState."RestoreVelocity") -> (queue out=w459:refnum<queue>)  [unwired: 2 in, 2 out]
          n174 = Enqueue Element At Opposite End(queue=w459, element=MeanderLoopState."Quit", error in (no error)=w469) -> (queue out=w465:refnum<queue>, error out=w466:errorcluster)  [unwired: 1 in, 1 out]
          n175 = Enqueue Element At Opposite End(queue=w465, element=MeanderLoopState."StopLaser", error in (no error)=w466) -> (error out=w464:errorcluster)  [unwired: 1 in, 2 out]
          n176 = Enqueue Element At Opposite End(queue=w468, element=T6 {"State"=enum."STOP", "Params."=variant}, error in (no error)=w464) -> ()  [unwired: 1 in, 3 out]
        }
        frame "Pause" {
          # "Not mature, skip"
          # "Stop stage, laser\nwait\nrestart stage, laser / Quit"
          n177 = while {
            shift-right: [w479] -> w475
            shift-left: w477 -> [w489]
            shift-right: [w481] -> w473
            shift-left: w474 -> [w490]
            stop <- w483 stop-if-true
            n178 = Preview Queue Element(queue=w490, timeout in ms (-1)=0, error in (no error)=w489) -> (queue out=w482:refnum<queue>, element=w487:T5, timed out?=w485:bool, error out=w484:errorcluster)
            n179 = call <userlib>:"Wait (ms)__ogtk.vi"("error in (no error)"=w484, "milliseconds to wait"=u32 200) -> ("error out"=w480:errorcluster)  [unwired: 8 in, 1 out]
            n180 = Equal?(x=MeanderLoopState."Pause", y=w487) -> (x = y?=w486:bool)
            n181 = Compound Arithmetic op=AND(w486, invert w485) -> (w483:bool)
            n182 = case shown="True" w483 {
              tunnel: w482 -> [w493 w497]
              tunnel: [w493 w496] -> w481
              tunnel: w480 -> [w492 w495]
              tunnel: [w492 w494] -> w479
              frame False {
              }
              frame True {
                n183 = Dequeue Element(queue=w497, error in (no error)=w495) -> (queue out=w496:refnum<queue>, error out=w494:errorcluster)  [unwired: 1 in, 2 out]
              }
            }
          }
          n184 = One Button Dialog(message="Internal error. Unexpected pause frame.") -> ()  [unwired: 1 in, 1 out]
          n185 = Enqueue Element At Opposite End(queue=w473, element=MeanderLoopState."StartOfLine", error in (no error)=w475) -> (error out=w476:errorcluster)  [unwired: 1 in, 2 out]
        }
        frame "Quit" {
          w499 = FALSE
          # "<= Just mark quit, so that restore high velocity can get the information."
        }
      }
      n186 = call <userlib>:"ErrorLog.vi"("error in (no error)"=w57) -> ("error out"=w47:errorcluster)  [unwired: 10 in]
      "InnerIter." <- w49
    }
  }
  "Interupted" <- w16
  n187 = while {
    tunnel: "AppsRef" -> [w504]
    tunnel: w12 -> [w501]
    stop <- w502 stop-if-true
    # "Interrupted Stop"
    n188 = Dequeue Element(queue=w504) -> (element=w503:T4)  [unwired: 2 in, 3 out]
    n189 = case shown="\"Interrupted_Stop\"" w503 {
      tunnel: [_ FALSE TRUE] -> w502
      tunnel: w501 -> [_ w507 _]
      frame Default {
      }
      frame "Interrupted_Stop" {
        n190 = Enqueue Element At Opposite End(queue=w507, element=MeanderLoopState."Exit", timeout in ms (-1)=1000) -> ()  [unwired: 1 in, 3 out]
      }
      frame "Quit_SubProgram" {
      }
    }
  }
  n191 = Increment(x=w22) -> (x+1=→"Actual_Line#":i32)
  n192 = Unbundle By Name(w3) -> ("Feedback"=w4:refnum<queue>)
  n193 = Unbundle By Name("QueuesRef") -> ("InfoRef"=w19:refnum<vi>)
  n194 = Release Queue(queue=w4, error in (no error)=w1) -> (error out=w2:errorcluster)  [unwired: 1 in, 2 out]
  n195 = property class="Str"(reference=w19, error in=w2, "Value"="") -> (error out=w13:errorcluster)  [unwired: 1 out]
  n196 = Release Queue(queue=w12, error in (no error)=w13) -> (error out=w11:errorcluster)  [unwired: 1 in, 2 out]
  n197 = Enqueue Element(queue="AppsRef", element=States-AToF."Quit_SubProgram", error in (no error)=w11) -> (error out=→"error out":errorcluster)  [unwired: 1 in, 2 out]
